vi "extra q palindrome using subset.vi"() -> ()   [LabVIEW 2025]
panel:
  in  "string":string
  out "is palindrome":bool
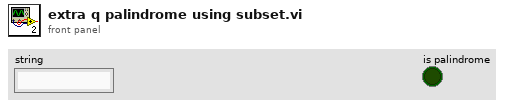
[diagram p1: front panel]
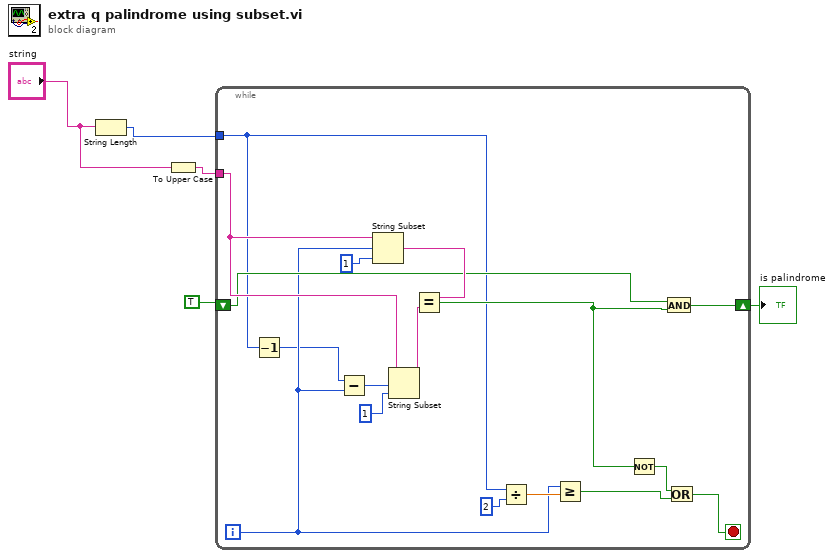
[diagram p0: block diagram]
diagram:
  n1 = String Length(string="string") -> (length=w1:i32)
  n2 = To Upper Case(1:"string") -> (0:w4:string)
  n3 = while {
    tunnel: w4 -> [w22]
    shift-right: [w15] -> w5
    shift-left: TRUE -> [w17]
    tunnel: w1 -> [w8]
    i -> [w9]
    stop <- w13 stop-if-true
    n4 = Decrement(x=w8) -> (x-1=w7:i32)
    n5 = Subtract(x=w7, y=w9) -> (x-y=w20:i32)
    n6 = String Subset(string=w22, offset (0)=w9, length (rest)=1) -> (substring=w19:string)
    n7 = String Subset(string=w22, offset (0)=w20, length (rest)=1) -> (substring=w18:string)
    n8 = Equal?(x=w19, y=w18) -> (x = y?=w16:bool)
    n9 = Divide(x=w8, y=2) -> (x/y=w11:dbl)
    n10 = Greater Or Equal?(x=w9, y=w11) -> (x >= y?=w10:bool)
    n11 = Not(x=w16) -> (.not. x?=w14:bool)
    n12 = And(x=w17, y=w16) -> (x .and. y?=w15:bool)
    n13 = Or(x=w14, y=w10) -> (x .or. y?=w13:bool)
  }
  "is palindrome" <- w5
